vi "Initialize.vi"(8 "error in (no error)":errorcluster, 11 "Board in":refnum<class "Board.lvclass">) -> (0 "error out":errorcluster, 3 "Board out":refnum<class "Board.lvclass">)   [LabVIEW 2015, in "TronviewGame.lvlib" / "Board.lvclass"]
uses:
  Board.lvclass
  FieldState.ctl
  Position.ctl
  Board.lvclass/Board.ctl
  GetBoardCenter.vi
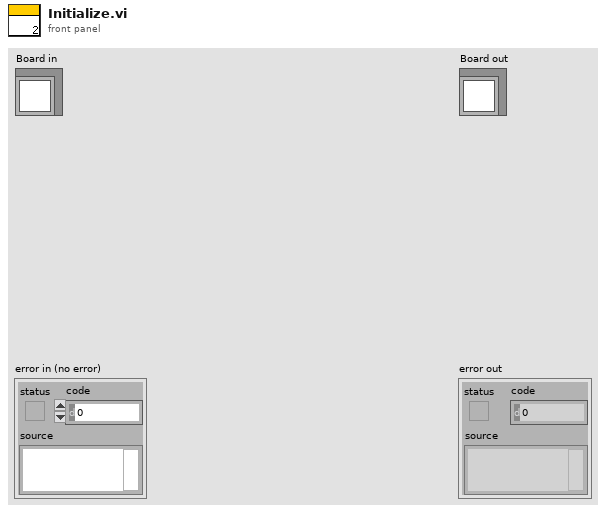
[diagram p1: front panel]
types:
  T1 = typedef "TronviewGame.lvlib/Board.lvclass/Position.ctl" = cluster{"Column":i32, "Row":i32}
  T2 = typedef "TronviewGame.lvlib/Board.lvclass/FieldState.ctl" = enum16{"Empty", "Blocked", "Player1Position", "Player2Postion", "Player1Marked", "Player2Marked"}
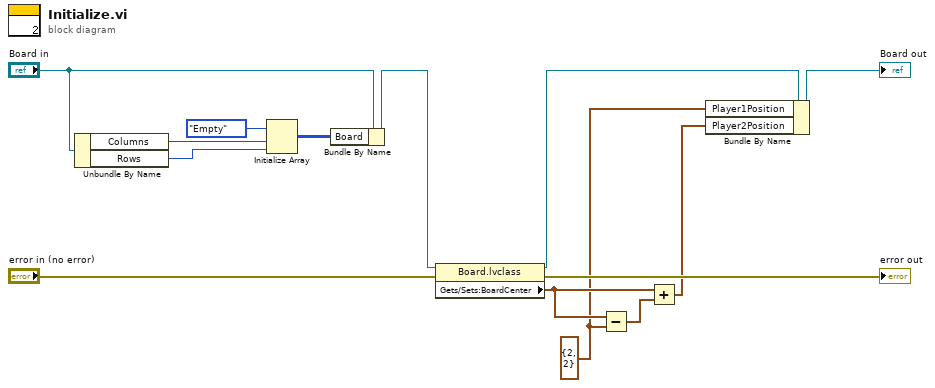
[diagram p0: block diagram]
diagram:
  w3 = T1 {"Column"=2, "Row"=2} ("Position")
  n1 = Unbundle By Name("Board in") -> ("Columns"=w9:u32, "Rows"=w12:u32)
  n2 = Initialize Array(FieldState."Empty" ("FieldState"), w9, w12) -> (w10:T2[][])
  n3 = Bundle By Name(cluster="Board in", "Board"=w10) -> (w7:refnum<class "Board.lvclass">)
  n4 = property class="Board.lvclass"(reference=w7, error in="error in (no error)") -> (reference out=w6:refnum<class "Board.lvclass">, error out=→"error out":errorcluster, "Gets/Sets:BoardCenter"=w5:T1)
  n5 = Subtract(x=w5, y=w3) -> (x-y=w2:T1)
  n6 = Add(x=w5, y=w2) -> (x+y=w1:T1)
  n7 = Bundle By Name(cluster=w6, "Player1Position"=w3, "Player2Position"=w1) -> (→"Board out":refnum<class "Board.lvclass">)
